vi "TestRunVI.vi"(11 "CLI input parameters":string[](array[string])) -> (2 "Message to log to console":string, 3 "exit code":i32)   [LabVIEW 2018]
uses:
  <vilib>/Utility/error.llb/DialogType.ctl
panel:
  out "element":string
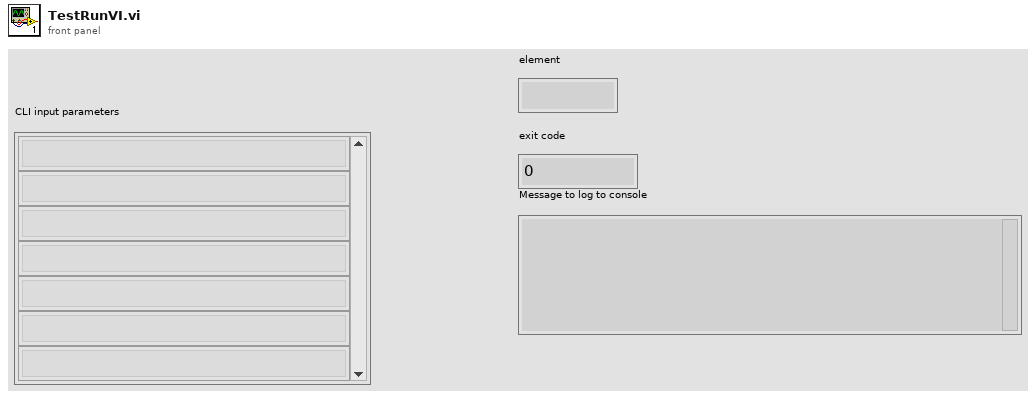
[diagram p1: front panel]
types:
  T1 = typedef "DialogType.ctl" = u16
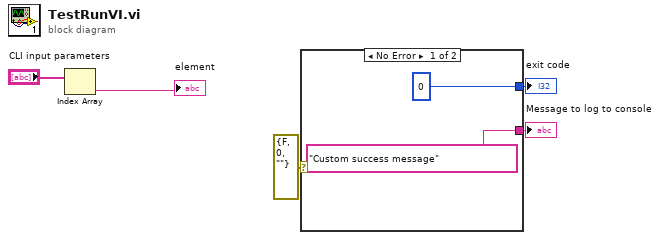
[diagram p0: block diagram]
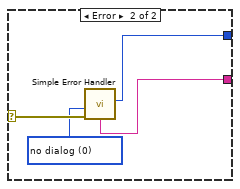
[diagram p2: hidden frame]
diagram:
  n1 = Index Array(array="CLI input parameters") -> (element=→"element":string)  [unwired: 1 in]
  n2 = case shown="No Error" errorcluster {"status"=FALSE, "code"=0, "source"=""} ("error IO") {
    selector: errorcluster {"status"=FALSE, "code"=0, "source"=""} ("error IO") -> [_ w11]
    tunnel: [0 ("exit code") w9] -> w5
    tunnel: ["Custom success message" w8] -> w4
    frame No Error {
    }
    frame Error {
      w10 = T1 0 items=["no dialog", "OK message", "continue or stop message", "OK message + warnings", "continue/stop + warnings"] ("type of dialog (OK msg:1)")
      n3 = call <vilib>:"Simple Error Handler.vi"("type of dialog (OK msg:1)"=w10, "error in (no error)"=w11) -> ("code out"=w9:i32, "message"=w8:string)  [unwired: 3 in, 3 out]
    }
  }
  "exit code" <- w5
  "Message to log to console" <- w4
